vi "FTP Get Whole Directory.vi"(8 "timeout ms (60000)":i32=200, 10 "Local Folder of Autonomous Plays":path, 11 "host":string="10.26.14.21") -> (0 "error out":errorcluster)   [LabVIEW 2015]
uses:
  <vilib>/FTP/ftp2.llb/FTP File Info.ctl
  <vilib>/FTP/NI_FTP.lvlib
panel:
  out "Non-matching file\nextension removed":T1[](array[typedef])
  in  "directory path":string="/Autonomous-Plays"
  in  "password":string
  in  "user":string="anonymous"
  out "file errors":errorcluster[](array[cluster])
  out "Converted DIR Specifications":T2(array[cluster])
  out "Raw dir list":T1[](array[typedef])
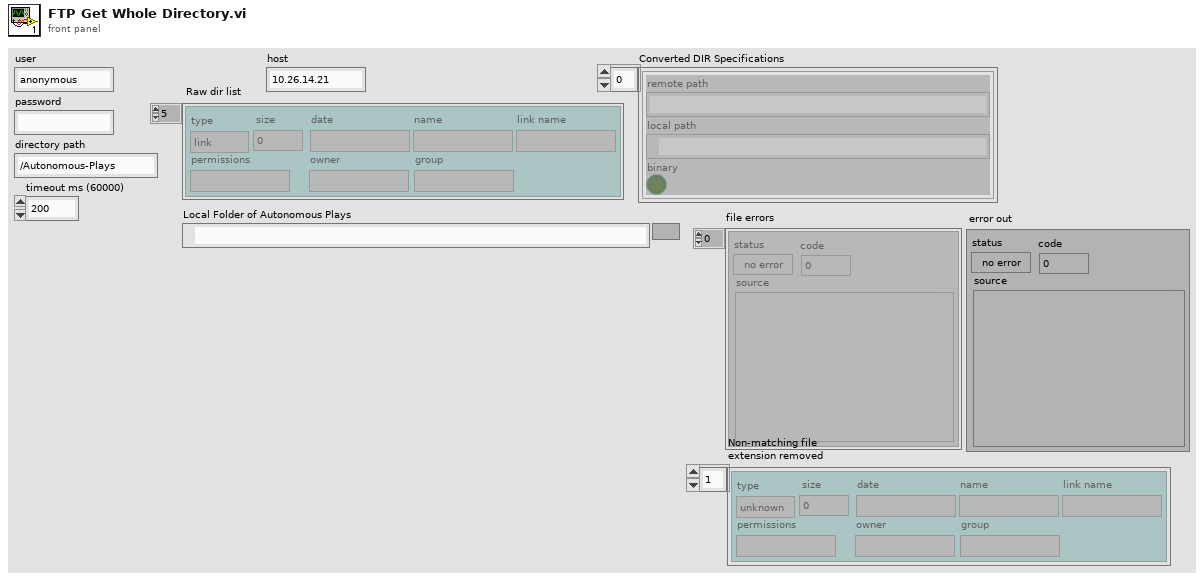
[diagram p1: front panel]
types:
  T1 = typedef "NI_FTP.lvlib/FTP File Info.ctl" = cluster{"type":enum16{"unknown", "file", "dir", "link"}, "permissions":string, "owner":string, "group":string, "size":i32, "date":string, "name":string, "link name":string}
  T2 = cluster{"remote path":string, "local path":path, "binary":bool}[]
  T3 = typedef "NI_FTP.lvlib/FTP Session.ctl" = refnum<k5>
  T4 = cluster{"remote path":string, "local path":path, "binary":bool}
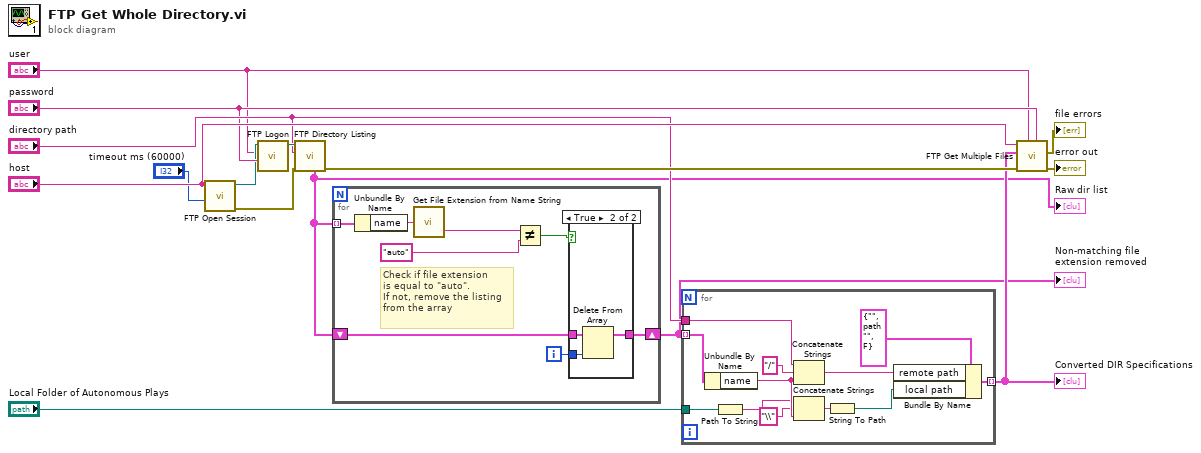
[diagram p0: block diagram]
diagram:
  n1 = call <vilib>:"FTP Open Session.vi"("timeout ms (60000)"="timeout ms (60000)", "address"="host") -> ("error out"=w15:errorcluster, "ftp session"=w5:T3)  [unwired: 6 in, 2 out]
  n2 = call <vilib>:"FTP Logon.vi"("password"="password", "user"="user", "ftp session"=w5) -> ("ftp session out"=w14:T3)  [unwired: 5 in, 3 out]
  n3 = call <vilib>:"FTP Directory Listing.vi"("error in (no error)"=w15, "directory path"="directory path", "ftp session"=w14) -> ("error out"=w12:errorcluster, "dir list"=w3:T1[])  [unwired: 4 in, 3 out]
  "Raw dir list" <- w3
  n4 = for {
    tunnel: w3 -> [w23] mode=indexing
    shift-right: [w17] -> w2
    shift-left: w3 -> [w20]
    i -> [w18]
    # "Check if file extension\nis equal to \"auto\".\nIf not, remove the listing\nfrom the array"
    n5 = Unbundle By Name(w23) -> ("name"=w22:string)
    n6 = call "Get File Extension from Name String.vi"("File Name String"=w22) -> ("lowercase file extension"=w16:string)  [unwired: 1 out]
    n7 = Not Equal?(x=w16, y="auto") -> (x != y?=w19:bool)
    n8 = case shown="True" w19 {
      tunnel: w20 -> [w24 w27]
      tunnel: w18 -> [_ w26]
      tunnel: [w24 w25] -> w17
      frame False {
      }
      frame True {
        n9 = Delete From Array(array=w27, index=w26) -> (array with subset deleted=w25:T1[])  [unwired: 1 in, 1 out]
      }
    }
  }
  "Non-matching file\nextension removed" <- w2
  n10 = for {
    tunnel: "directory path" -> [w39]
    tunnel: "Local Folder of Autonomous Plays" -> [w35]
    tunnel: [w36] -> w9 mode=indexing
    tunnel: w2 -> [w28] mode=indexing
    n11 = Unbundle By Name(w28) -> ("name"=w34:string)
    n12 = Path To String(path=w35) -> (string=w32:string)
    n13 = Concatenate Strings(w39, "/" ("string"), w34) -> (w38:string)
    n14 = Concatenate Strings(w32, "\\" ("string"), w34) -> (w30:string)
    n15 = String To Path(string=w30) -> (path=w31:path)
    n16 = Bundle By Name(cluster=T4 {"remote path"="", "local path"=path "", "binary"=FALSE} ("transfer spec"), "remote path"=w38, "local path"=w31) -> (w36:T4)
  }
  "Converted DIR Specifications" <- w9
  n17 = call <vilib>:"FTP Get Multiple Files.vi"("password"="password", "user"="user", "error in (no error)"=w12, "file specifications"=w9, "host"="host") -> ("error out"=→"error out":errorcluster, "file errors"=→"file errors":errorcluster[])  [unwired: 5 in]
